vi "CCD Acquire Spectrum vs Wavelength Range Mode.vi"() -> ()   [LabVIEW 2020, in "Examples.lvlib"]
doc: "Example for a CCD spectrum acquisition."
uses:
  Examples.lvlib
  Classes/CCD/CCD.lvclass
  Classes/Mono/Monochromator.lvclass
  Mono/CCD Wavelength Range Mode Enum.ctl
  1eaaf627-5626-46cd-b4c0-03ad69b9d17c.vi
  c61b53c0-740b-458e-9fea-2d818d683ba3.vi
  b5b558cd-b5a0-42ff-a173-51559e4ee0fb.vi
  78a3a600-9171-4017-88e3-26cc5737fe19.vi
  f9a36742-f95e-48a9-8e85-5b022f2dda12.vi
  6683dd4e-dda6-4711-a464-d3489a04f865.vi
  a4719100-13a0-4dba-b2b8-8abdf787bee2.vi
  d9dcfbd1-fdc5-46d0-ab02-778f704a0cfe.vi
  b2b273e1-28ce-414c-878a-ce11b2a339d7.vi
  24bc1878-ba86-4b2f-8076-166b862aba04.vi
  785b6cdc-67cc-4ea5-8f22-258210858afd.vi
  261f53a0-1808-4b57-ab80-f5aa02968533.vi
  8d1b6d21-e6aa-4ec1-a90b-49a40cb42e66.vi
  Classes/CCD/roiMetaData.ctl
  Classes/CCD/imageAcqData.ctl
  Classes/CCD/ccdAcquisitionData.ctl
panel:
  out "Intensity Graph 2":dbl[][](graph)
  out "XY Graph 2":T1(graph)
  out "error out":errorcluster
  in  "error in":errorcluster
  out "Intensity Graph":dbl[][](graph)
  out "XY Graph":T1(graph)
  in  "Stop Position Check 2":bool
  in  "Stop Slit Check":bool
  out "shutterPosition":i32
  out "shutterIndex":i32
  in  "Stop Position Check":bool
  in  "Stop Move Mirror Check":bool
  in  "Stop Grating Check":bool
  in  "Stop Init Check":bool
  out "Mono Initialized":bool
  # "Connector Pane"
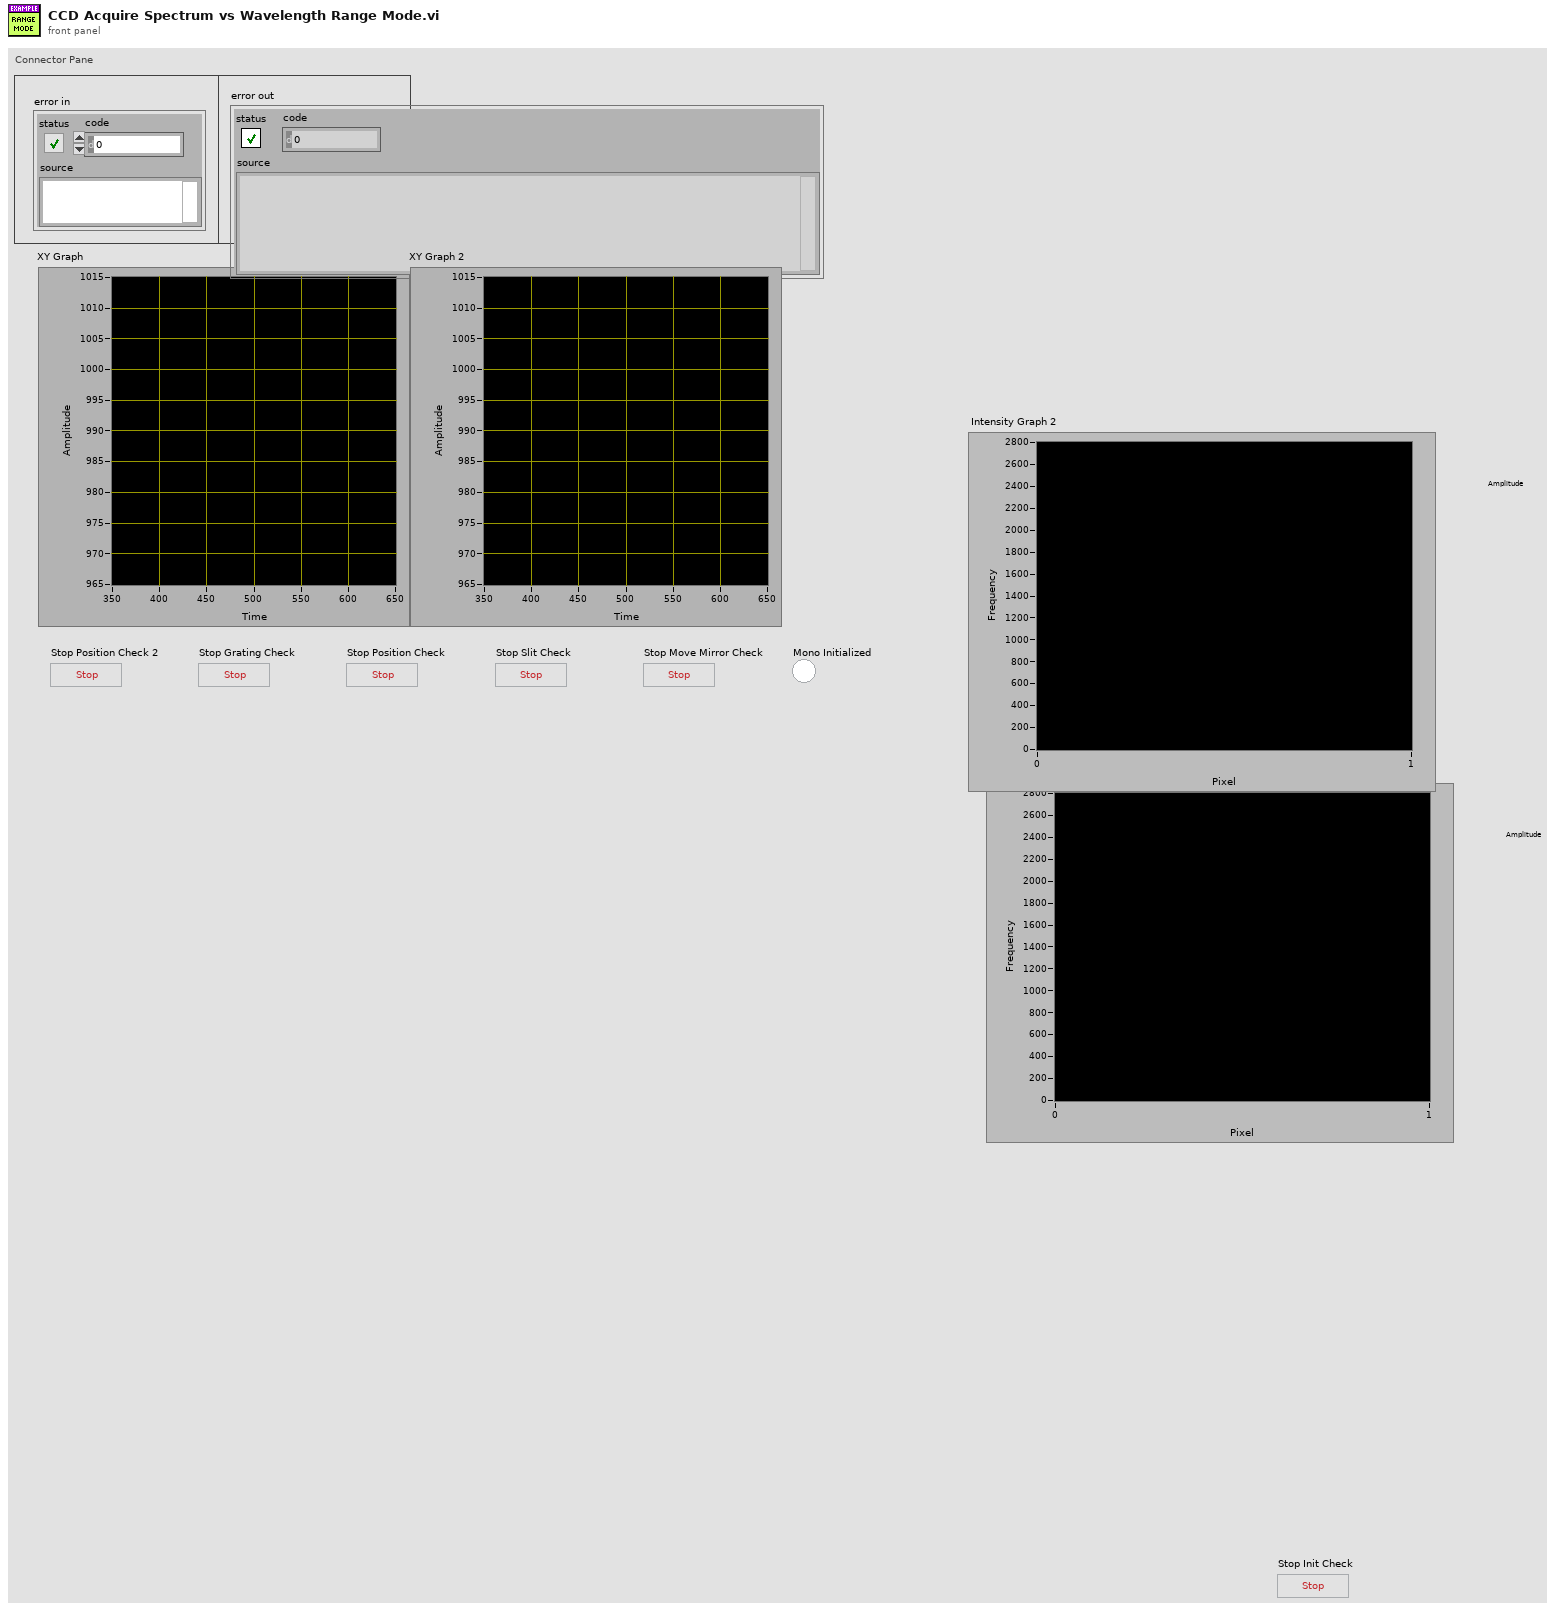
[diagram p1: front panel]
types:
  T1 = cluster{"Stitched Data Out":dbl[], "Stitched Data Out":dbl[]}
  T2 = typedef "horiba.lvlib/CCD.lvclass/ccdAcquisitionData.ctl" = cluster{"acqIndex":i32, "ROIs":T3[], "timestamp":string}
  T3 = typedef "horiba.lvlib/CCD.lvclass/imageAcqData.ctl" = cluster{"roiMetaData":T4, "xAxis":dbl[], "yData":dbl[][]}
  T4 = typedef "horiba.lvlib/CCD.lvclass/roiMetaData.ctl" = cluster{"roiIndex":i32, "xBinning":i32, "xOrigin":i32, "xSize":i32, "yBinning":i32, "yOrigin":i32, "ySize":i32}
  T5 = cluster{"startWavelength":dbl, "endWavelength":dbl, "Positions":dbl[], "ccdAcquisitions":T2[][]}
  T6 = typedef "CCD Wavelength Range Mode Enum.ctl" = enum16{"Open Device Manager", "Open Devices", "Initialize Mono", "Mono Settings", "Move Mono", "Camera Acquisition Settings", "Acquire Camera Data", "Data Processing", "Close Devices", "Close Device Manager"}
  T7 = cluster{"ROI-index":i32, "xOrigin":i32, "yOrigin":i32, "xSize":i32, "ySize":i32, "xBin":i32, "yBin":i32}
  T8 = cluster{"monoIndex":i32, "startWavelength":dbl, "endWavelength":dbl, "overlap":dbl}
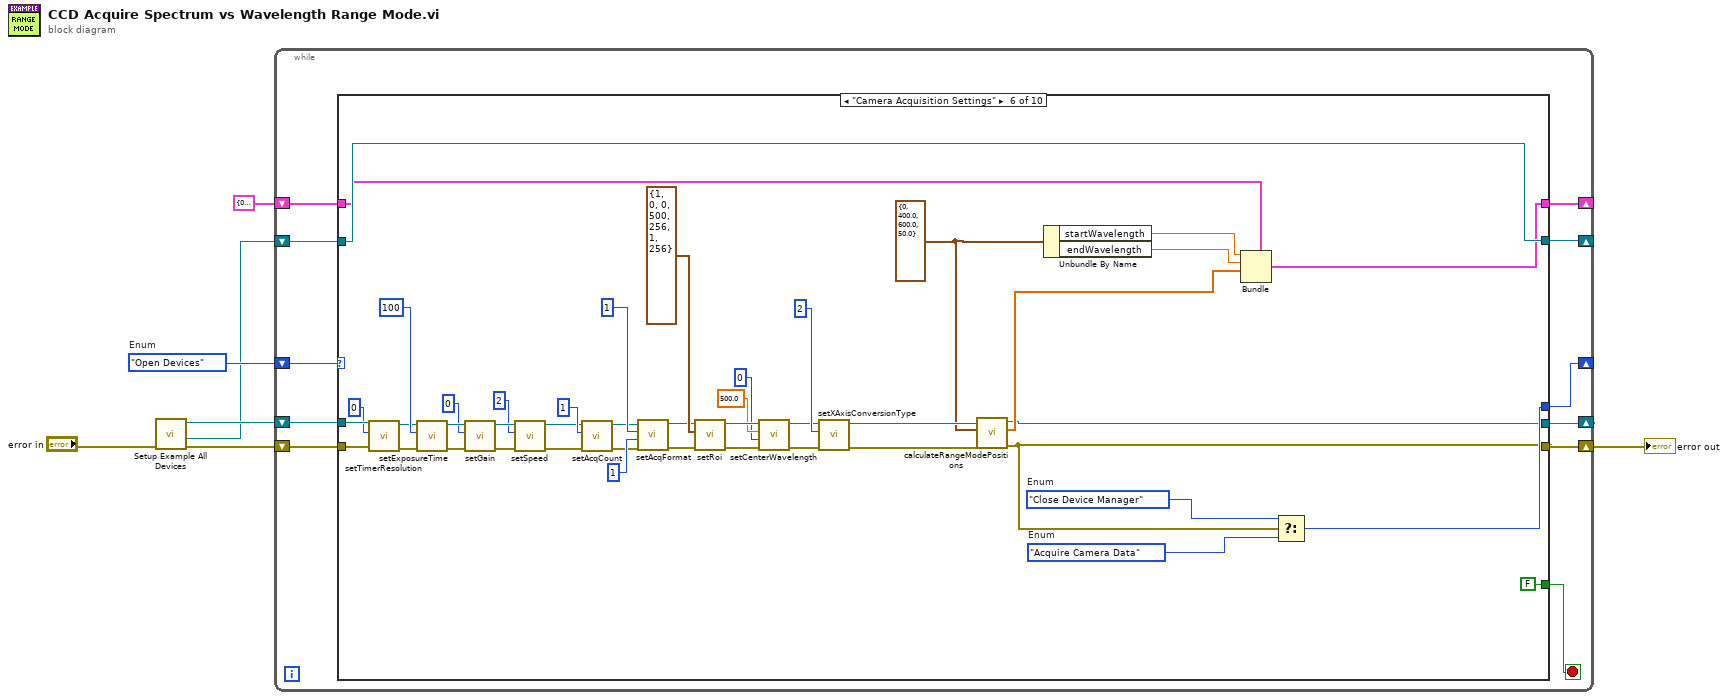
[diagram p0: block diagram]
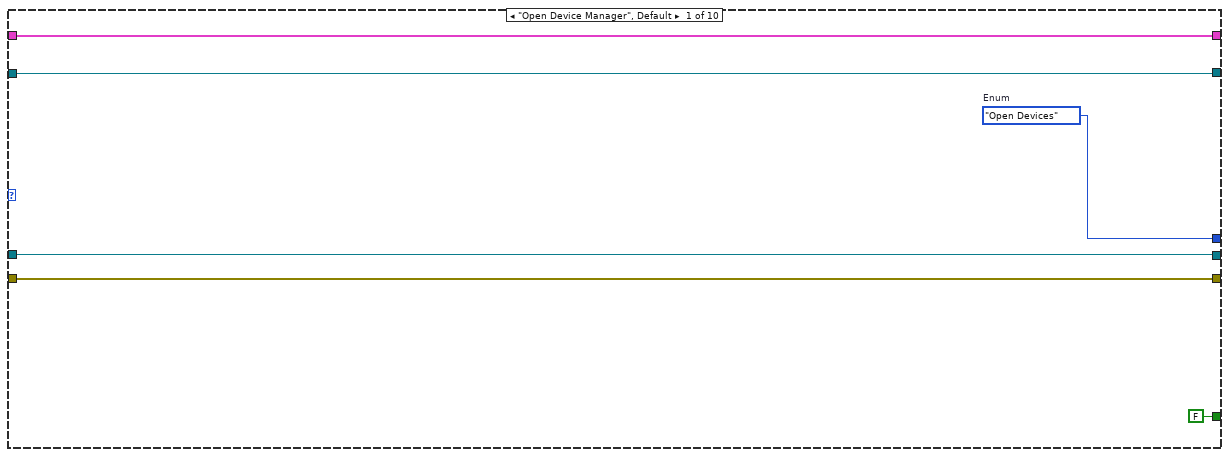
[diagram p2: hidden frame]
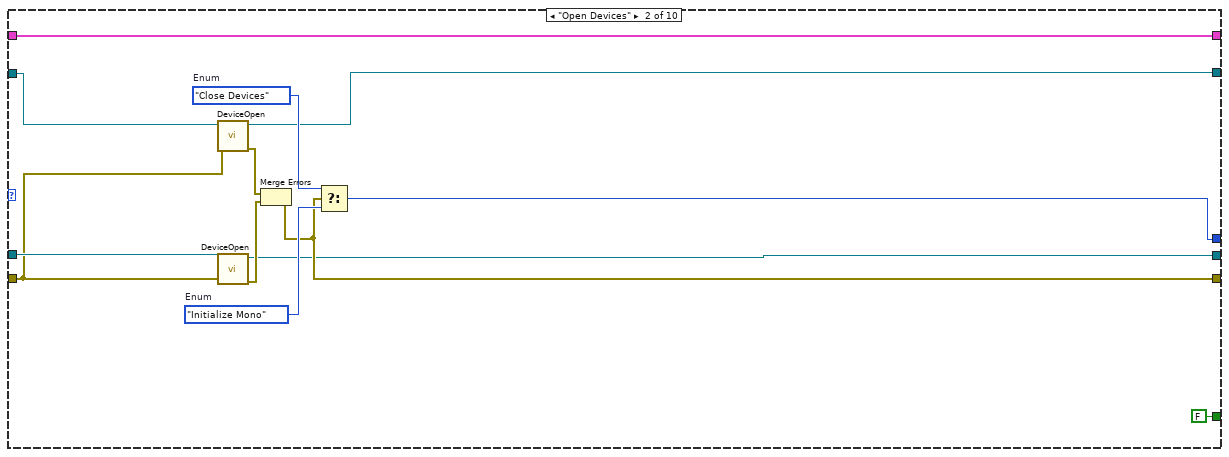
[diagram p3: hidden frame]
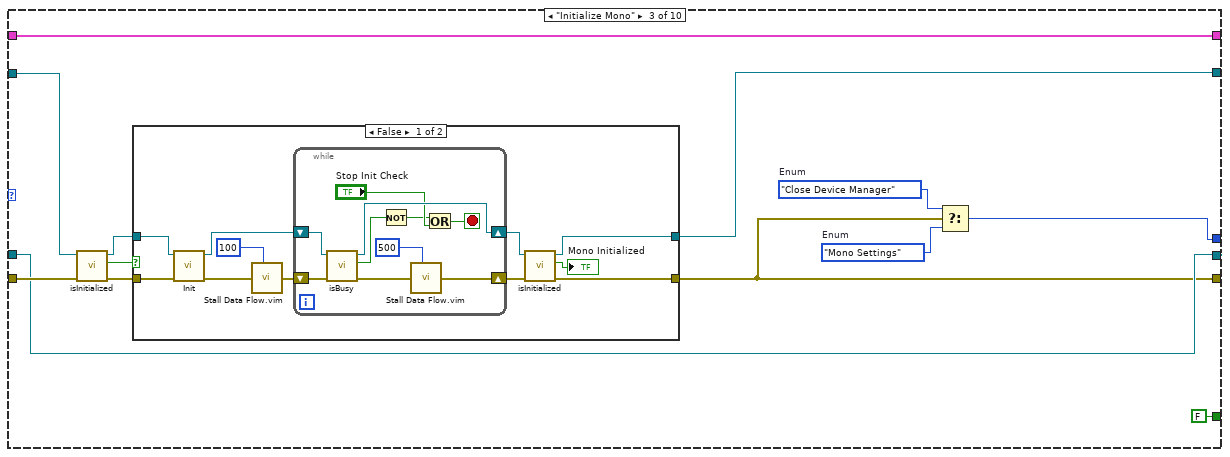
[diagram p4: hidden frame]
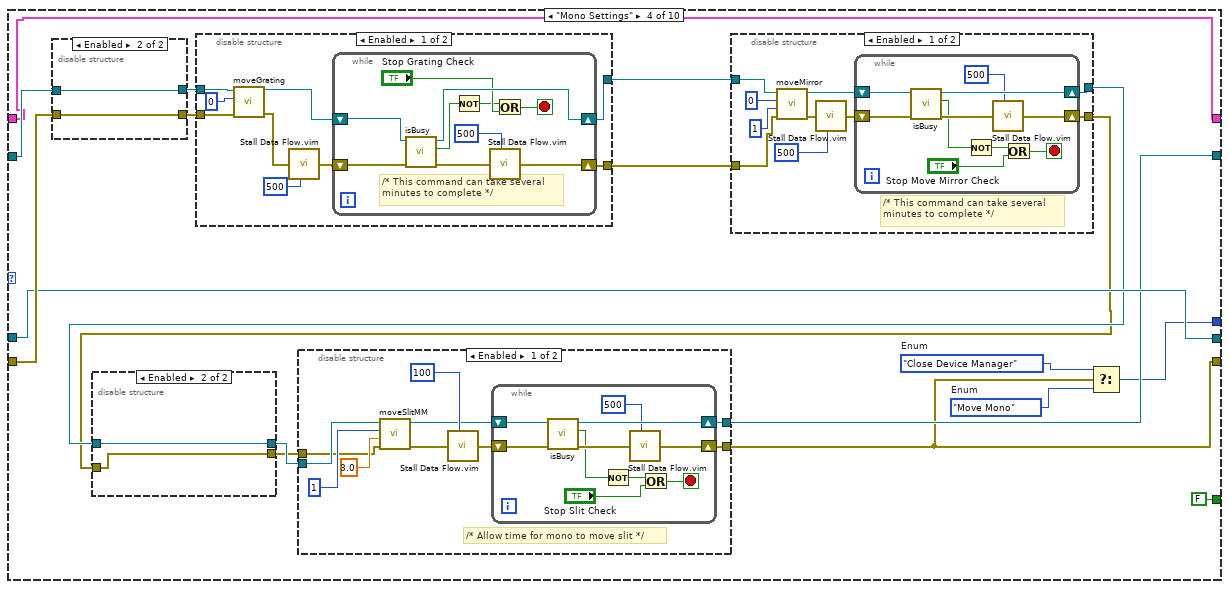
[diagram p6: hidden frame]
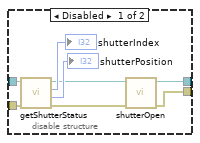
[diagram p8: hidden frame]
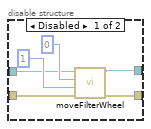
[diagram p11: hidden frame]
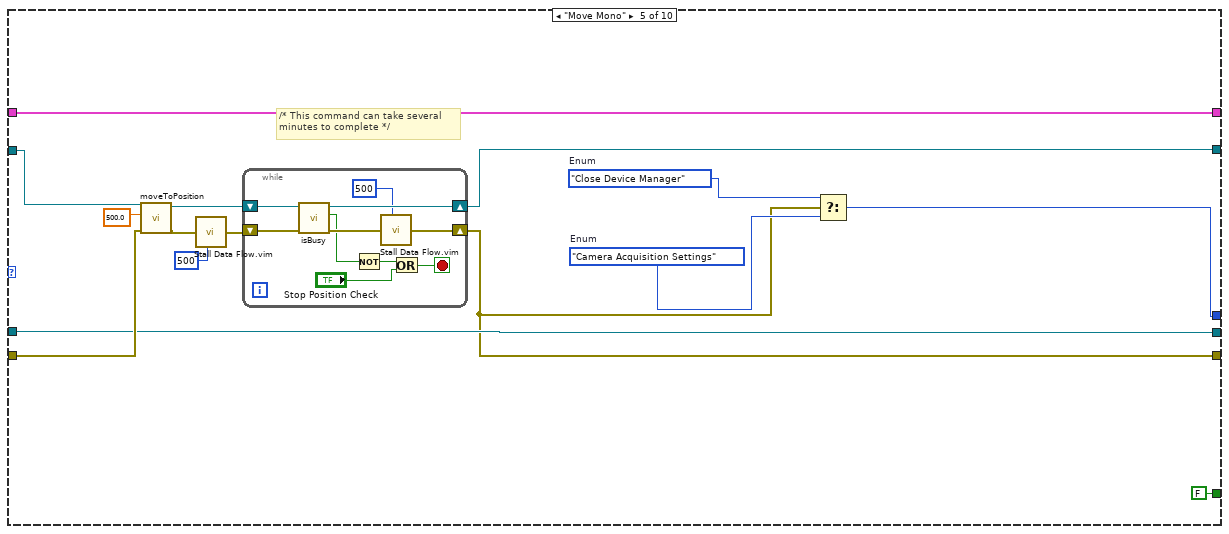
[diagram p12: hidden frame]
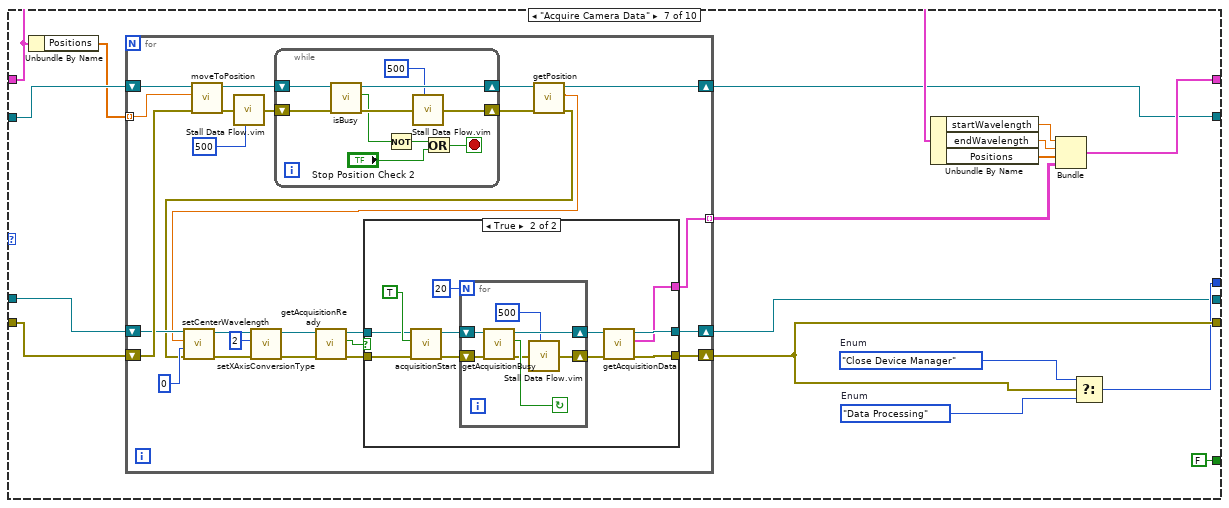
[diagram p13: hidden frame]
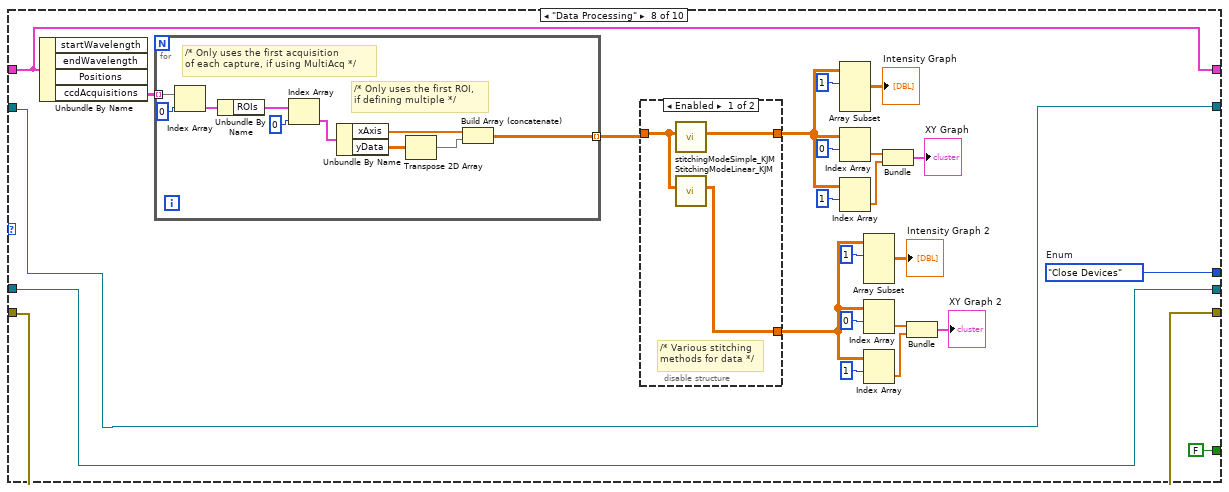
[diagram p15: hidden frame]
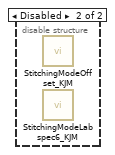
[diagram p16: hidden frame]
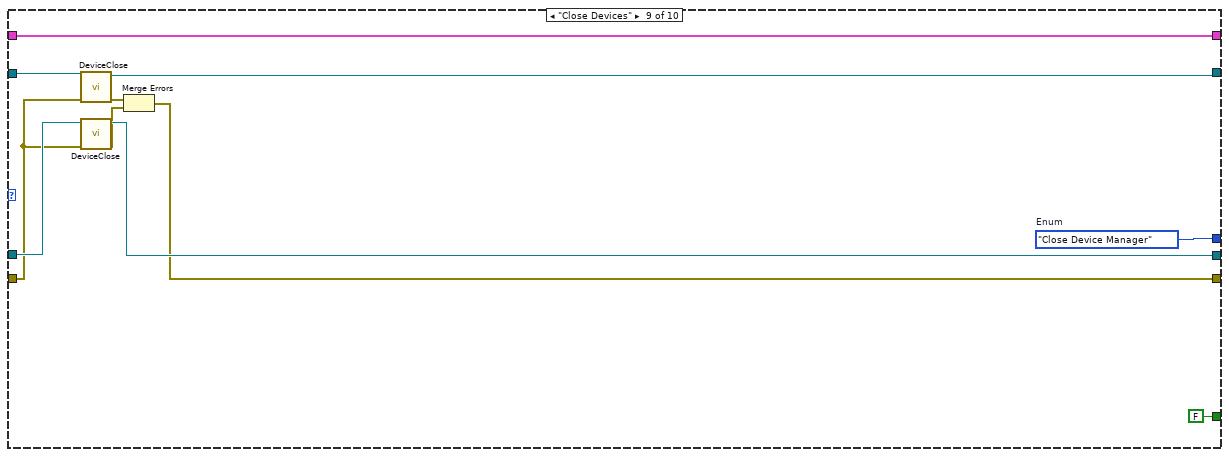
[diagram p17: hidden frame]
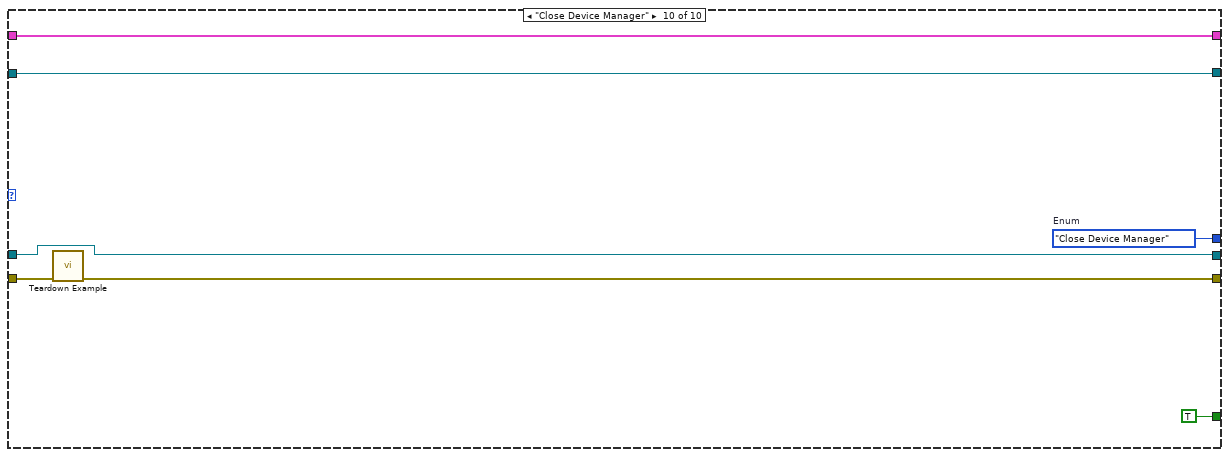
[diagram p18: hidden frame]
diagram:
  w7 = CCD_Wavelength_Range_Mode_Enum."Open Devices"  # Enum
  n1 = call "Setup Example All Devices.vi"("error in (no error)"="error in") -> ("error out"=w6:errorcluster, "Mono out"=w4:refnum<class "Monochromator.lvclass">, "CCD out"=w5:refnum<class "CCD.lvclass">)  [unwired: 6 in, 2 out]
  n2 = while {
    shift-right: [w14] -> w1
    shift-left: w6 -> [w17]
    shift-right: [w8] -> _
    shift-left: w7 -> [w18]
    shift-right: [w13] -> _
    shift-left: w4 -> [w15]
    shift-right: [w12] -> _
    shift-left: w5 -> [w16]
    shift-right: [w11] -> _
    shift-left: T5 {"startWavelength"=0.0, "endWavelength"=0.0, "Positions"=[], "ccdAcquisitions"=[]} -> [w10]
    stop <- w9 stop-if-true
    n3 = case shown="\"Camera Acquisition Settings\"" w18 {
      tunnel: w17 -> [w21 w35 w47 w90 w183 w225 w260 w327 w361 w370]
      tunnel: w16 -> [w22 w37 w44 w87 w181 w235 w244 w326 w362 w367]
      tunnel: w15 -> [w23 w36 w46 w91 w184 w208 w259 w325 w363 w366]
      tunnel: [w21 w30 w43 w78 w177 w214 w248 w327 w356 w369] -> w14
      tunnel: [w20 w29 w40 w75 w176 w215 w246 w331 w355 w364] -> w8
      tunnel: [FALSE FALSE FALSE FALSE FALSE FALSE FALSE FALSE FALSE TRUE] -> w9
      tunnel: [w23 w28 w45 w82 w182 w208 w251 w325 w359 w366] -> w13
      tunnel: [w22 w27 w44 w87 w181 w207 w245 w326 w360 w367] -> w12
      tunnel: [w24 w25 w38 w74 w175 w200 w252 w338 w353 w365] -> w11
      tunnel: w10 -> [w24 w25 w38 w74 w175 w201 w257 w338 w353 w365]
      frame "Open Device Manager", Default {
        w20 = CCD_Wavelength_Range_Mode_Enum."Open Devices"  # Enum
      }
      frame "Open Devices" {
        w31 = CCD_Wavelength_Range_Mode_Enum."Initialize Mono"  # Enum
        w32 = CCD_Wavelength_Range_Mode_Enum."Close Devices"  # Enum
        n4 = call-dynamic "DeviceOpen.vi"("error in (no error)"=w35, "Monochromator in"=w36) -> ("error out"=w33:errorcluster, "Monochromator out"=w28:refnum<class "Monochromator.lvclass">)  [unwired: 6 in, 2 out]
        n5 = call-dynamic "DeviceOpen.vi"("error in (no error)"=w35, "CCD in"=w37) -> ("error out"=w34:errorcluster, "CCD out"=w27:refnum<class "CCD.lvclass">)  [unwired: 6 in, 2 out]
        n6 = Merge Errors(w33, w34) -> (w30:errorcluster)
        n7 = Select(t=w32, s=w30, f=w31) -> (s? t:f=w29:T6)
      }
      frame "Initialize Mono" {
        w41 = CCD_Wavelength_Range_Mode_Enum."Close Device Manager"  # Enum
        w42 = CCD_Wavelength_Range_Mode_Enum."Mono Settings"  # Enum
        n8 = call "isInitialized.vi"("error in (no error)"=w47, "Monochromator in"=w46) -> ("error out"=w49:errorcluster, "mono is initialized?"=w50:bool, "Monochromator out"=w48:refnum<class "Monochromator.lvclass">)  [unwired: 7 in]
        n9 = case shown="False" w50 {
          tunnel: [w59 w73] -> w43
          tunnel: [w58 w72] -> w45
          tunnel: w49 -> [w52 w73]
          tunnel: w48 -> [w51 w72]
          frame False {
            n10 = call "Init.vi"("error in (no error)"=w52, "Monochromator in"=w51) -> ("error out"=w61:errorcluster, "Monochromator out"=w60:refnum<class "Monochromator.lvclass">)  [unwired: 6 in, 2 out]
            n11 = call "Stall Data Flow.vim"("value in"=w61, "milliseconds to wait"=u32 100) -> ("value out"=w56:errorcluster)  [unwired: 1 out]
            n12 = while {
              shift-right: [w67] -> w54
              shift-left: w56 -> [w69]
              shift-right: [w70] -> w55
              shift-left: w60 -> [w68]
              stop <- w64 stop-if-true
              n13 = call "isBusy.vi"("error in (no error)"=w69, "Monochromator in"=w68) -> ("error out"=w71:errorcluster, "mono is busy?"=w65:bool, "Monochromator out"=w70:refnum<class "Monochromator.lvclass">)  [unwired: 7 in]
              n14 = Not(x=w65) -> (.not. x?=w62:bool)
              n15 = call "Stall Data Flow.vim"("value in"=w71, "milliseconds to wait"=u32 500) -> ("value out"=w67:errorcluster)  [unwired: 1 out]
              n16 = Or(x=w62, y="Stop Init Check") -> (x .or. y?=w64:bool)
            }
            n17 = call "isInitialized.vi"("error in (no error)"=w54, "Monochromator in"=w55) -> ("error out"=w59:errorcluster, "mono is initialized?"=→"Mono Initialized":bool, "Monochromator out"=w58:refnum<class "Monochromator.lvclass">)  [unwired: 7 in]
          }
          frame True {
          }
        }
        n18 = Select(t=w41, s=w43, f=w42) -> (s? t:f=w40:T6)
      }
      frame "Mono Settings" {
        w76 = CCD_Wavelength_Range_Mode_Enum."Move Mono"  # Enum
        w77 = CCD_Wavelength_Range_Mode_Enum."Close Device Manager"  # Enum
        n19 = disable-structure shown="Enabled" {
          disable-tunnel: w91 -> [w170 w174]
          disable-tunnel: w90 -> [w169 w173]
          disable-tunnel: [w168 w173] -> w89
          disable-tunnel: [w167 w174] -> w88
          frame Disabled {
            n20 = call "moveFilterWheel.vi"("error in (no error)"=w169, "position"=1, "locationId"=0, "Monochromator in"=w170) -> ("error out"=w168:errorcluster, "Monochromator out"=w167:refnum<class "Monochromator.lvclass">)  [unwired: 4 in, 2 out]
          }
          frame Enabled {
          }
        }
        n21 = disable-structure shown="Enabled" {
          disable-tunnel: w89 -> [w149 w165]
          disable-tunnel: w88 -> [w148 w166]
          disable-tunnel: [w147 w166] -> w86
          disable-tunnel: [w146 w165] -> w85
          frame Enabled {
            n22 = call "moveGrating.vi"("error in (no error)"=w149, "position"=0, "Monochromator in"=w148) -> ("error out"=w154:errorcluster, "Monochromator out"=w152:refnum<class "Monochromator.lvclass">)  [unwired: 5 in, 2 out]
            n23 = call "Stall Data Flow.vim"("value in"=w154, "milliseconds to wait"=u32 500) -> ("value out"=w153:errorcluster)  [unwired: 1 out]
            n24 = while {
              shift-right: [w160] -> w146
              shift-left: w153 -> [w162]
              shift-right: [w163] -> w147
              shift-left: w152 -> [w161]
              stop <- w157 stop-if-true
              # "/* This command can take several \nminutes to complete */"
              n25 = call "isBusy.vi"("error in (no error)"=w162, "Monochromator in"=w161) -> ("error out"=w164:errorcluster, "mono is busy?"=w158:bool, "Monochromator out"=w163:refnum<class "Monochromator.lvclass">)  [unwired: 7 in]
              n26 = Not(x=w158) -> (.not. x?=w155:bool)
              n27 = call "Stall Data Flow.vim"("value in"=w164, "milliseconds to wait"=u32 500) -> ("value out"=w160:errorcluster)  [unwired: 1 out]
              n28 = Or(x=w155, y="Stop Grating Check") -> (x .or. y?=w157:bool)
            }
          }
          frame Disabled {
          }
        }
        n29 = disable-structure shown="Enabled" {
          disable-tunnel: w86 -> [w127 w145]
          disable-tunnel: w85 -> [w126 w144]
          disable-tunnel: [w125 w145] -> w84
          disable-tunnel: [w124 w144] -> w81
          frame Enabled {
            # "/* This command can take several \nminutes to complete */"
            n30 = call "moveMirror.vi"("error in (no error)"=w126, "position"=1, "locationId"=0, "Monochromator in"=w127) -> ("error out"=w132:errorcluster, "Monochromator out"=w129:refnum<class "Monochromator.lvclass">)  [unwired: 4 in, 2 out]
            n31 = call "Stall Data Flow.vim"("value in"=w132, "milliseconds to wait"=u32 500) -> ("value out"=w131:errorcluster)  [unwired: 1 out]
            n32 = while {
              shift-right: [w139] -> w124
              shift-left: w131 -> [w141]
              shift-right: [w142] -> w125
              shift-left: w129 -> [w140]
              stop <- w136 stop-if-true
              n33 = call "isBusy.vi"("error in (no error)"=w141, "Monochromator in"=w140) -> ("error out"=w143:errorcluster, "mono is busy?"=w137:bool, "Monochromator out"=w142:refnum<class "Monochromator.lvclass">)  [unwired: 7 in]
              n34 = Not(x=w137) -> (.not. x?=w134:bool)
              n35 = call "Stall Data Flow.vim"("value in"=w143, "milliseconds to wait"=u32 500) -> ("value out"=w139:errorcluster)  [unwired: 1 out]
              n36 = Or(x=w134, y="Stop Move Mirror Check") -> (x .or. y?=w136:bool)
            }
          }
          frame Disabled {
          }
        }
        n37 = disable-structure shown="Enabled" {
          disable-tunnel: w84 -> [w117 w123]
          disable-tunnel: [w116 w123] -> w83
          disable-tunnel: w81 -> [w115 w122]
          disable-tunnel: [w114 w122] -> w80
          frame Disabled {
            n38 = call "getShutterStatus.vi"("error in (no error)"=w115, "Monochromator in"=w117) -> ("error out"=w118:errorcluster, "shutterPosition"=→"shutterPosition":i32, "shutterIndex"=→"shutterIndex":i32, "Monochromator out"=w119:refnum<class "Monochromator.lvclass">)  [unwired: 6 in]
            n39 = call "shutterOpen.vi"("error in (no error)"=w118, "Monochromator in"=w119) -> ("error out"=w114:errorcluster, "Monochromator out"=w116:refnum<class "Monochromator.lvclass">)  [unwired: 6 in, 2 out]
          }
          frame Enabled {
          }
        }
        n40 = disable-structure shown="Enabled" {
          disable-tunnel: w83 -> [w95 w112]
          disable-tunnel: [w94 w112] -> w82
          disable-tunnel: w80 -> [w93 w113]
          disable-tunnel: [w92 w113] -> w78
          frame Enabled {
            # "/* Allow time for mono to move slit */"
            n41 = call "moveSlitMM.vi"("error in (no error)"=w93, "position"=3.0, "locationId"=1, "Monochromator in"=w95) -> ("error out"=w101:errorcluster, "Monochromator out"=w96:refnum<class "Monochromator.lvclass">)  [unwired: 4 in, 2 out]
            n42 = call "Stall Data Flow.vim"("value in"=w101, "milliseconds to wait"=u32 100) -> ("value out"=w97:errorcluster)  [unwired: 1 out]
            n43 = while {
              shift-right: [w107] -> w92
              shift-left: w97 -> [w109]
              shift-right: [w110] -> w94
              shift-left: w96 -> [w108]
              stop <- w104 stop-if-true
              n44 = call "isBusy.vi"("error in (no error)"=w109, "Monochromator in"=w108) -> ("error out"=w111:errorcluster, "mono is busy?"=w105:bool, "Monochromator out"=w110:refnum<class "Monochromator.lvclass">)  [unwired: 7 in]
              n45 = Not(x=w105) -> (.not. x?=w102:bool)
              n46 = call "Stall Data Flow.vim"("value in"=w111, "milliseconds to wait"=u32 500) -> ("value out"=w107:errorcluster)  [unwired: 1 out]
              n47 = Or(x=w102, y="Stop Slit Check") -> (x .or. y?=w104:bool)
            }
          }
          frame Disabled {
          }
        }
        n48 = Select(t=w77, s=w78, f=w76) -> (s? t:f=w75:T6)
      }
      frame "Move Mono" {
        w178 = CCD_Wavelength_Range_Mode_Enum."Close Device Manager"  # Enum
        w179 = CCD_Wavelength_Range_Mode_Enum."Camera Acquisition Settings"  # Enum
        # "/* This command can take several \nminutes to complete */"
        n49 = call "moveToPosition.vi"("error in (no error)"=w183, "wavelength"=500.0, "Monochromator in"=w184) -> ("error out"=w186:errorcluster, "Monochromator out"=w188:refnum<class "Monochromator.lvclass">)  [unwired: 5 in, 2 out]
        n50 = call "Stall Data Flow.vim"("value in"=w186, "milliseconds to wait"=u32 500) -> ("value out"=w187:errorcluster)  [unwired: 1 out]
        n51 = while {
          shift-right: [w195] -> w177
          shift-left: w187 -> [w197]
          shift-right: [w198] -> w182
          shift-left: w188 -> [w196]
          stop <- w192 stop-if-true
          n52 = call "isBusy.vi"("error in (no error)"=w197, "Monochromator in"=w196) -> ("error out"=w199:errorcluster, "mono is busy?"=w193:bool, "Monochromator out"=w198:refnum<class "Monochromator.lvclass">)  [unwired: 7 in]
          n53 = Not(x=w193) -> (.not. x?=w190:bool)
          n54 = call "Stall Data Flow.vim"("value in"=w199, "milliseconds to wait"=u32 500) -> ("value out"=w195:errorcluster)  [unwired: 1 out]
          n55 = Or(x=w190, y="Stop Position Check") -> (x .or. y?=w192:bool)
        }
        n56 = Select(t=w178, s=w177, f=w179) -> (s? t:f=w176:T6)
      }
      frame "Camera Acquisition Settings" {
        w212 = T8 {"monoIndex"=0, "startWavelength"=400.0, "endWavelength"=600.0, "overlap"=50.0} ("calculateRangeModePositions")
        w242 = CCD_Wavelength_Range_Mode_Enum."Close Device Manager"  # Enum
        w243 = CCD_Wavelength_Range_Mode_Enum."Acquire Camera Data"  # Enum
        n57 = call "setTimerResolution.vi"("error in (no error)"=w225, "resolutionToken"=0, "CCD in"=w235) -> ("error out"=w224:errorcluster, "CCD out"=w234:refnum<class "CCD.lvclass">)  [unwired: 5 in, 2 out]
        n58 = call "setExposureTime.vi"("error in (no error)"=w224, "exposure time [ms] or [us]"=100, "CCD in"=w234) -> ("error out"=w223:errorcluster, "CCD out"=w233:refnum<class "CCD.lvclass">)  [unwired: 5 in, 2 out]
        n59 = call "setGain.vi"("error in (no error)"=w223, "token"=0, "CCD in"=w233) -> ("error out"=w222:errorcluster, "CCD out"=w232:refnum<class "CCD.lvclass">)  [unwired: 5 in, 2 out]
        n60 = call "setSpeed.vi"("error in (no error)"=w222, "token"=2, "CCD in"=w232) -> ("error out"=w221:errorcluster, "CCD out"=w231:refnum<class "CCD.lvclass">)  [unwired: 5 in, 2 out]
        n61 = call "setAcqCount.vi"("error in (no error)"=w221, "count"=1, "CCD in"=w231) -> ("error out"=w220:errorcluster, "CCD out"=w230:refnum<class "CCD.lvclass">)  [unwired: 5 in, 2 out]
        n62 = call "setAcqFormat.vi"("error in (no error)"=w220, "format"=1, "number of ROIs"=1, "CCD in"=w230) -> ("error out"=w219:errorcluster, "CCD out"=w229:refnum<class "CCD.lvclass">)  [unwired: 4 in, 2 out]
        n63 = call "setRoi.vi"("error in (no error)"=w219, "roiConfig"=T7 {"ROI-index"=1, "xOrigin"=0, "yOrigin"=0, "xSize"=500, "ySize"=256, "xBin"=1, "yBin"=256}, "CCD in"=w229) -> ("error out"=w218:errorcluster, "CCD out"=w228:refnum<class "CCD.lvclass">)  [unwired: 5 in, 2 out]
        n64 = call "setCenterWavelength.vi"("error in (no error)"=w218, "monoIndex"=0, "wavelength"=500.0, "CCD in"=w228) -> ("error out"=w217:errorcluster, "CCD out"=w227:refnum<class "CCD.lvclass">)  [unwired: 4 in, 2 out]
        n65 = call "setXAxisConversionType.vi"("error in (no error)"=w217, "type"=2, "CCD in"=w227) -> ("error out"=w216:errorcluster, "CCD out"=w226:refnum<class "CCD.lvclass">)  [unwired: 5 in, 2 out]
        n66 = call "calculateRangeModePositions.vi"("error in (no error)"=w216, "calculateRangeModePositions"=w212, "CCD in"=w226) -> ("error out"=w214:errorcluster, "Positions"=w211:dbl[], "CCD out"=w207:refnum<class "CCD.lvclass">)  [unwired: 5 in, 1 out]
        n67 = Unbundle By Name(w212) -> ("startWavelength"=w209:dbl, "endWavelength"=w210:dbl)
        n68 = Bundle(cluster=w201, "startWavelength"=w209, "endWavelength"=w210, "Positions"=w211) -> (w200:T5)  [unwired: 1 in]
        n69 = Select(t=w242, s=w214, f=w243) -> (s? t:f=w215:T6)
      }
      frame "Acquire Camera Data" {
        w249 = CCD_Wavelength_Range_Mode_Enum."Close Device Manager"  # Enum
        w247 = CCD_Wavelength_Range_Mode_Enum."Data Processing"  # Enum
        n70 = Unbundle By Name(w257) -> ("Positions"=w258:dbl[])
        n71 = for {
          tunnel: w258 -> [w276] mode=indexing
          shift-right: [w270] -> w248
          shift-left: w260 -> [w274]
          shift-right: [w269] -> w245
          shift-left: w244 -> [w268]
          shift-right: [w262] -> w251
          shift-left: w259 -> [w275]
          tunnel: [w267] -> w253 mode=indexing
          n72 = call "moveToPosition.vi"("error in (no error)"=w274, "wavelength"=w276, "Monochromator in"=w275) -> ("error out"=w283:errorcluster, "Monochromator out"=w285:refnum<class "Monochromator.lvclass">)  [unwired: 5 in, 2 out]
          n73 = call "Stall Data Flow.vim"("value in"=w283, "milliseconds to wait"=u32 500) -> ("value out"=w284:errorcluster)  [unwired: 1 out]
          n74 = while {
            shift-right: [w311] -> w264
            shift-left: w284 -> [w313]
            shift-right: [w314] -> w265
            shift-left: w285 -> [w312]
            stop <- w308 stop-if-true
            n75 = call "isBusy.vi"("error in (no error)"=w313, "Monochromator in"=w312) -> ("error out"=w315:errorcluster, "mono is busy?"=w309:bool, "Monochromator out"=w314:refnum<class "Monochromator.lvclass">)  [unwired: 7 in]
            n76 = Not(x=w309) -> (.not. x?=w306:bool)
            n77 = call "Stall Data Flow.vim"("value in"=w315, "milliseconds to wait"=u32 500) -> ("value out"=w311:errorcluster)  [unwired: 1 out]
            n78 = Or(x=w306, y="Stop Position Check 2") -> (x .or. y?=w308:bool)
          }
          n79 = call "getPosition.vi"("error in (no error)"=w264, "Monochromator in"=w265) -> ("error out"=w263:errorcluster, "wavelength"=w261:dbl, "Monochromator out"=w262:refnum<class "Monochromator.lvclass">)  [unwired: 7 in]
          n80 = call "setCenterWavelength.vi"("error in (no error)"=w263, "monoIndex"=0, "wavelength"=w261, "CCD in"=w268) -> ("error out"=w278:errorcluster, "CCD out"=w280:refnum<class "CCD.lvclass">)  [unwired: 4 in, 2 out]
          n81 = call "setXAxisConversionType.vi"("error in (no error)"=w278, "type"=2, "CCD in"=w280) -> ("error out"=w277:errorcluster, "CCD out"=w279:refnum<class "CCD.lvclass">)  [unwired: 5 in, 2 out]
          n82 = call "getAcquisitionReady.vi"("error in (no error)"=w277, "CCD in"=w279) -> ("error out"=w271:errorcluster, "ready"=w273:bool, "CCD out"=w272:refnum<class "CCD.lvclass">)  [unwired: 7 in]
          n83 = case shown="True" w273 {
            tunnel: [w286 w293] -> w270
            tunnel: [w287 w291] -> w269
            tunnel: [_ w290] -> w267
            tunnel: w272 -> [w287 w289]
            tunnel: w271 -> [w286 w288]
            frame False {
            }
            frame True {
              n84 = call "acquisitionStart.vi"("error in (no error)"=w288, "openShutter"=TRUE, "CCD in"=w289) -> ("error out"=w295:errorcluster, "CCD out"=w294:refnum<class "CCD.lvclass">)  [unwired: 5 in, 2 out]
              n85 = for {
                N: 20 -> [_]
                shift-right: [w301] -> w296
                shift-left: w295 -> [w304]
                shift-right: [w300] -> w292
                shift-left: w294 -> [w305]
                stop <- w303 continue-if-true
                n86 = call "getAcquisitionBusy.vi"("error in (no error)"=w304, "CCD in"=w305) -> ("error out"=w302:errorcluster, "isBusy"=w303:bool, "CCD out"=w300:refnum<class "CCD.lvclass">)  [unwired: 7 in]
                n87 = call "Stall Data Flow.vim"("value in"=w302, "milliseconds to wait"=u32 500) -> ("value out"=w301:errorcluster)  [unwired: 1 out]
              }
              n88 = call "getAcquisitionData.vi"("error in (no error)"=w296, "CCD in"=w292) -> ("error out"=w293:errorcluster, "ccdAcquisitions"=w290:T2[], "CCD out"=w291:refnum<class "CCD.lvclass">)  [unwired: 6 in, 1 out]
            }
          }
        }
        n89 = Unbundle By Name(w257) -> ("startWavelength"=w256:dbl, "endWavelength"=w255:dbl, "Positions"=w254:dbl[])
        n90 = Bundle("startWavelength"=w256, "endWavelength"=w255, "Positions"=w254, "ccdAcquisitions"=w253) -> (w252:T5)  [unwired: 1 in]
        n91 = Select(t=w249, s=w248, f=w247) -> (s? t:f=w246:T6)
      }
      frame "Data Processing" {
        w331 = CCD_Wavelength_Range_Mode_Enum."Close Devices"  # Enum
        n92 = Unbundle By Name(w338) -> ("ccdAcquisitions"=w339:T2[][])  [unwired: 3 out]
        n93 = for {
          tunnel: w339 -> [w352] mode=indexing
          tunnel: [w345] -> w324 mode=indexing
          # "/* Only uses the first ROI, \nif defining multiple */"
          # "/* Only uses the first acquisition \nof each capture, if using MultiAcq */"
          n94 = Index Array(array=w352, index=0) -> (element=w351:T2)
          n95 = Unbundle By Name(w351) -> ("ROIs"=w350:T3[])
          n96 = Index Array(array=w350, index=0) -> (element=w347:T3)
          n97 = Unbundle By Name(w347) -> ("xAxis"=w343:dbl[], "yData"=w344:dbl[][])
          n98 = Transpose 2D Array(2D array=w344) -> (transposed array=w346:dbl[][])
          n99 = Build Array (concatenate)(w343, w346) -> (w345:dbl[][])
        }
        n100 = disable-structure shown="Enabled" {
          disable-tunnel: [w342 _] -> w330
          disable-tunnel: w324 -> [w341 _]
          disable-tunnel: [w340 _] -> w316
          frame Enabled {
            # "/* Various stitching \nmethods for data */"
            n101 = call "stitchingModeSimple_KJM.vi"("Data In"=w341) -> ("Stitched Data Out"=w342:dbl[][])  [unwired: 9 in]
            n102 = call "StitchingModeLinear_KJM.vi"("Data In"=w341) -> ("Data Out"=w340:dbl[][])  [unwired: 9 in]
          }
          frame Disabled {
            n103 = call "StitchingModeOffset_KJM.vi"() -> ()  [unwired: 10 in, 1 out]
            n104 = call "StitchingModeLabspec6_KJM.vi"() -> ()  [unwired: 10 in, 1 out]
          }
        }
        n105 = Array Subset(array=w330, index (row)=1 ("index")) -> (→"Intensity Graph":dbl[][])  [unwired: 3 in]
        n106 = Index Array(array=w330, index (row)=0) -> (element=w335:dbl[])  [unwired: 1 in]
        n107 = Index Array(array=w330, index (row)=1 ("index")) -> (element=w333:dbl[])  [unwired: 1 in]
        n108 = Array Subset(array=w316, index (row)=1 ("index")) -> (→"Intensity Graph 2":dbl[][])  [unwired: 3 in]
        n109 = Index Array(array=w316, index (row)=0) -> (element=w322:dbl[])  [unwired: 1 in]
        n110 = Index Array(array=w316, index (row)=1 ("index")) -> (element=w320:dbl[])  [unwired: 1 in]
        n111 = Bundle("Stitched Data Out"=w335, "Stitched Data Out"=w333) -> (→"XY Graph":T1)  [unwired: 1 in]
        n112 = Bundle("Data Out"=w322, "Data Out"=w320) -> (→"XY Graph 2":cluster{"Data Out":dbl[], "Data Out":dbl[]})  [unwired: 1 in]
      }
      frame "Close Devices" {
        w355 = CCD_Wavelength_Range_Mode_Enum."Close Device Manager"  # Enum
        n113 = call-dynamic "DeviceClose.vi"("error in (no error)"=w361, "Monochromator in"=w363) -> ("error out"=w358:errorcluster, "Monochromator out"=w359:refnum<class "Monochromator.lvclass">)  [unwired: 5 in, 3 out]
        n114 = call-dynamic "DeviceClose.vi"("error in (no error)"=w361, "CCD in"=w362) -> ("error out"=w357:errorcluster, "CCD out"=w360:refnum<class "CCD.lvclass">)  [unwired: 5 in, 3 out]
        n115 = Merge Errors(w358, w357) -> (w356:errorcluster)
      }
      frame "Close Device Manager" {
        w364 = CCD_Wavelength_Range_Mode_Enum."Close Device Manager"  # Enum
        n116 = call "Teardown Example.vi"("error in (no error)"=w370) -> ("error out"=w369:errorcluster)  [unwired: 10 in]
      }
    }
  }
  "error out" <- w1
